vi "CopiaDeCopiaPAI.vi"() -> ()   [LabVIEW 2024]
uses:
  <vilib>/MakerHub/LINX/LMH-LINX.lvlib
  <vilib>/MakerHub/LINX/Public/Peripherals/Digital/Digital Read 1 Chan.vi
  <vilib>/MakerHub/LINX/Public/Peripherals/Digital/Digital Write 1 Chan.vi
  <vilib>/MakerHub/LINX/Public/Utilities/Open Serial.vi
panel:
  in  "Tab Control":enum32{"Inicio", "Sistema"}(tab)
  in  "Open Button 2":bool
  in  "Contraseña":string
  in  "Usuario":string
  out "Led 1":bool
  out "Led 2":bool
  out "Led 3":bool
  out "Led 4":bool
  out "Led 5":bool
  out "Pin2":dbl
  out "Pin3":dbl
  out "Pin4":dbl
  out "Pin5":dbl
  out "Pin6":dbl
  in  "Puerto Serial":refnum<visa-resource-name>="N/A"
  in  "Secuencia":dbl
  out "Contenido":dbl
  in  "Detener":bool
  in  "stop 4":bool
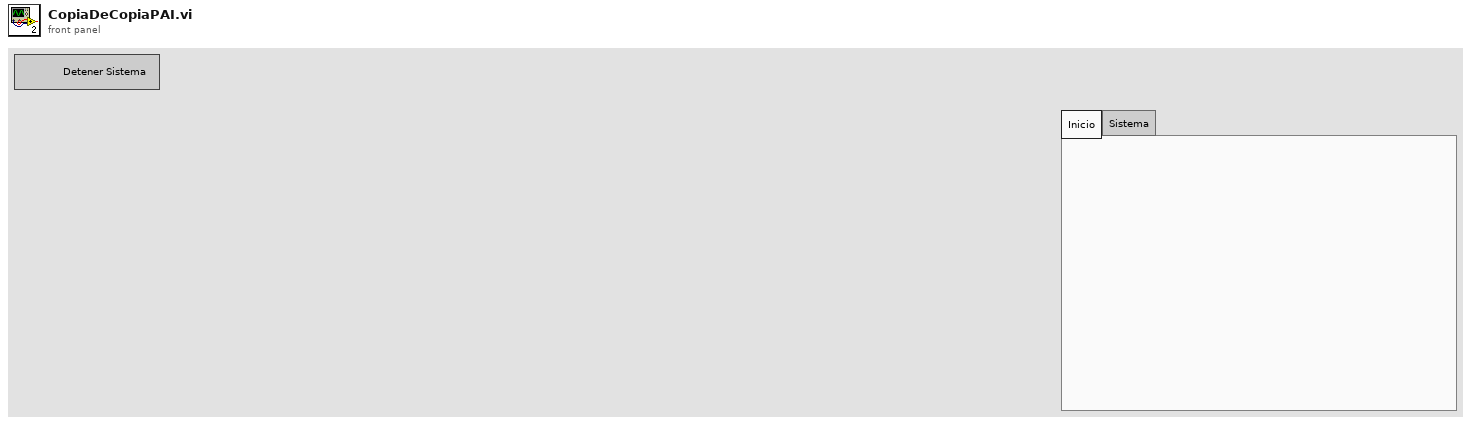
[diagram p1: front panel]
types:
  T1 = typedef "LMH-LINX.lvlib/LINX Ref.ctl" = cluster{"IO":T2, "Interface":T3, "LINX Device Config":T4}
  T2 = typedef "LMH-LINX.lvlib/Platform.ctl" = enum16{"Remote", "Local"}
  T3 = typedef "LMH-LINX.lvlib/Interface.ctl" = enum16{"Serial", "TCP"}
  T4 = typedef "LMH-LINX.lvlib/Device.lvlib/LINX Device Config.ctl" = cluster{"Interface":T3, "COM Port":refnum<visa-resource-name>, "TCP Configuration":T5, "Device Family":u8, "Device ID":u8, "Device Name":string, "TCP Ref":refnum<k5>, "Channels":T6}
  T5 = typedef "LMH-LINX.lvlib/Device.lvlib/TCP Config.ctl" = cluster{"IP Address":string, "Port":u16}
  T6 = typedef "LMH-LINX.lvlib/Channels.ctl" = cluster{"DI":u8[], "DO":u8[], "AI":u8[], "AO":u8[], "PWM":u8[], "QE":u8[], "UART":u8[], "I2C 2":u8[], "SPI":u8[], "CAN":u8[], "Servo":u8[], "AI Ref (V)":dbl, "AI Resolution (Bits)":u8, "AO Ref (V)":dbl, "AO Resolution (Bits)":u8}
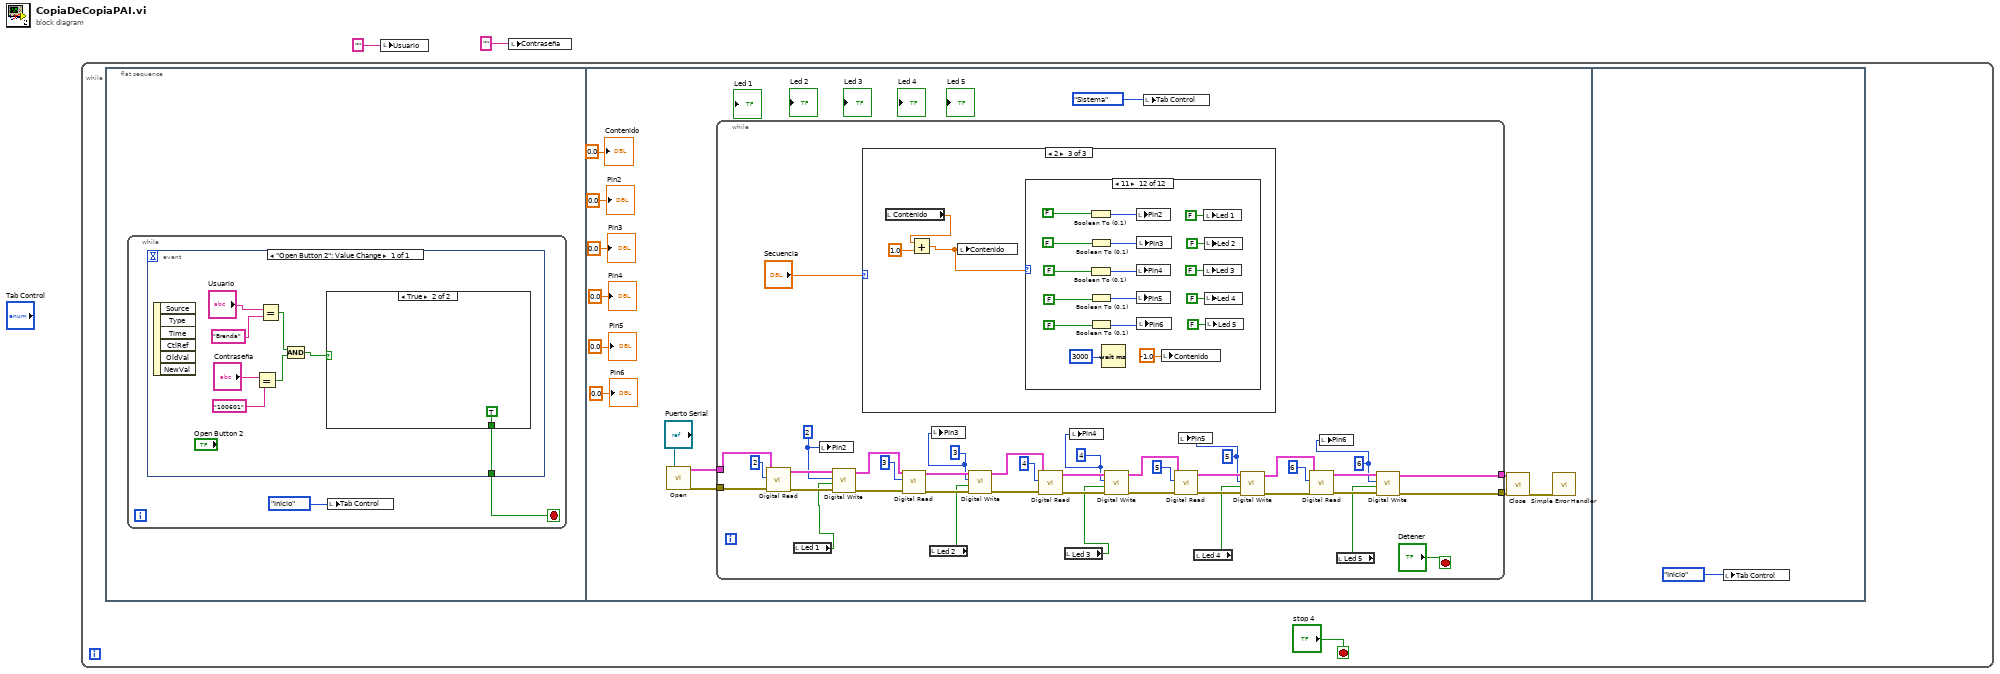
[diagram p0: block diagram]
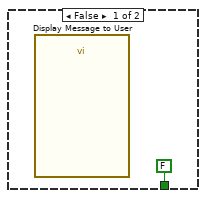
[diagram p2: hidden frame]
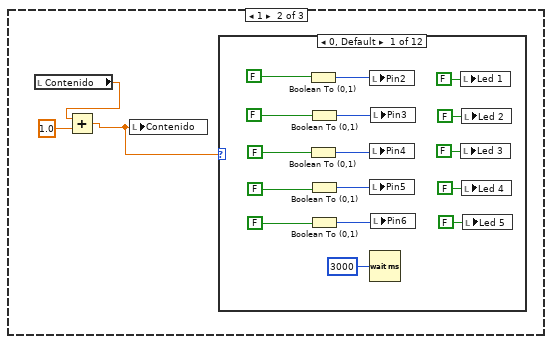
[diagram p4: hidden frame]
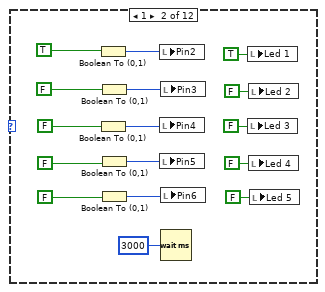
[diagram p5: hidden frame]
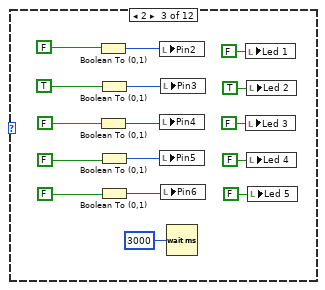
[diagram p6: hidden frame]
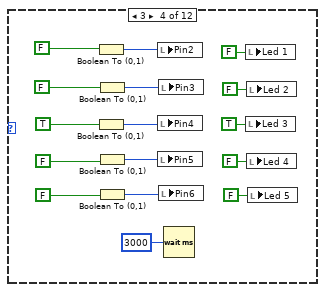
[diagram p7: hidden frame]
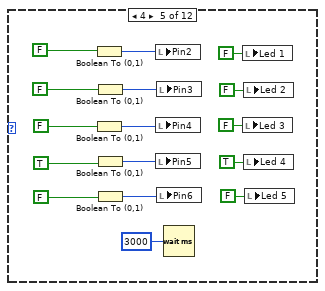
[diagram p8: hidden frame]
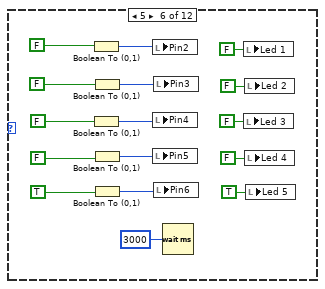
[diagram p9: hidden frame]
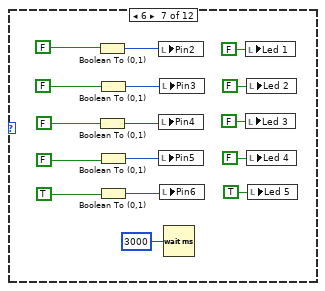
[diagram p10: hidden frame]
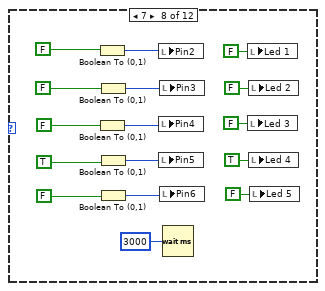
[diagram p11: hidden frame]
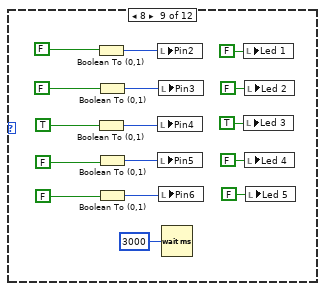
[diagram p12: hidden frame]
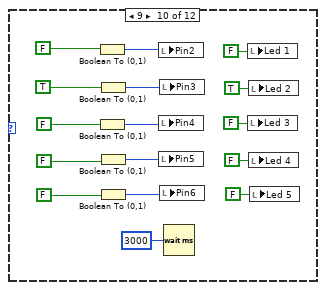
[diagram p13: hidden frame]
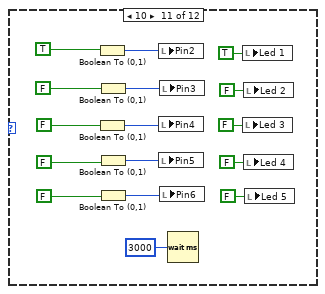
[diagram p14: hidden frame]
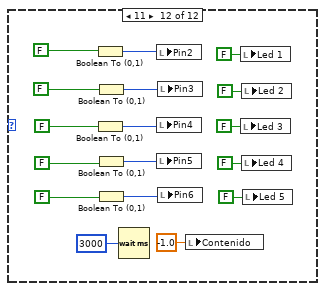
[diagram p15: hidden frame]
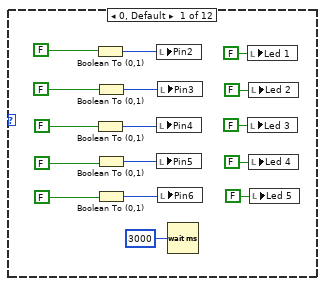
[diagram p16: hidden frame]
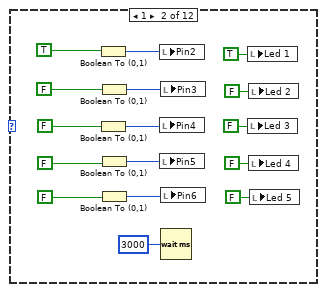
[diagram p17: hidden frame]
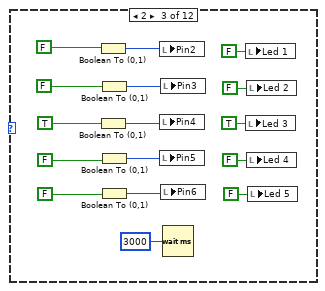
[diagram p18: hidden frame]
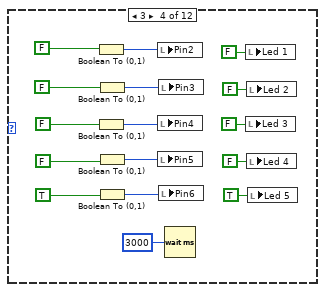
[diagram p19: hidden frame]
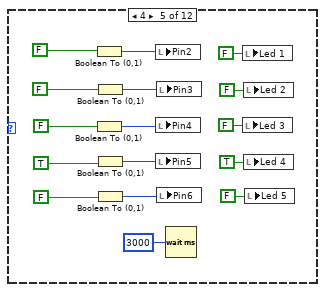
[diagram p20: hidden frame]
diagram:
  n1 = while {
    stop <- "stop 4" stop-if-true
    n2 = flat-sequence {
      frame #0 {
        n3 = while {
          stop <- w5 stop-if-true
          n4 = event shown="[0] \"Open Button 2\": Value Change" {
            selector: _ -> [_]
            dyn-events: _ -> [_]
            timeout: _ -> [_]
            tunnel: [w8] -> w5
            event "Open Button 2": Value Change {
              n5 = event-data() -> ()  [unwired: 1 in, 6 out]
              n6 = Equal?(x="Contraseña", y="100601") -> (x = y?=w10:bool)
              n7 = Equal?(x="Usuario", y="Brenda") -> (x = y?=w11:bool)
              n8 = And(x=w11, y=w10) -> (x .and. y?=w9:bool)
              n9 = case shown="True" w9 {
                tunnel: [FALSE TRUE] -> w8
                frame False {
                  n10 = call "Display Message to User"() -> ()  [unwired: 10 in, 2 out]
                }
                frame True {
                }
              }
            }
          }
          n11 = local write "Tab Control"(enum32{"Inicio", "Sistema"}."Inicio" ("Tab Control")) -> ()
        }
      }
      frame #1 {
        n12 = call-poly <vilib>:"Open.vi"("Serial Port"="Puerto Serial") -> ("Error Out"=w17:errorcluster, "LINX Resource"=w18:T1)  [unwired: 8 in, 1 out]
        n13 = while {
          tunnel: [w34] -> w20
          tunnel: [w33] -> w19
          tunnel: w18 -> [w32]
          tunnel: w17 -> [w31]
          stop <- "Detener" stop-if-true
          w35 = u8 6 ("DO Channel")
          w38 = u8 5 ("DO Channel")
          w39 = u8 4 ("DO Channel")
          w44 = u8 3 ("DO Channel")
          w42 = u8 2 ("DO Channel")
          n14 = call-poly <vilib>:"Digital Read.vi"("Error In"=w31, "DI Channel"=u8 2, "LINX Resource"=w32) -> ("Error Out"=w53:errorcluster, "LINX Resource"=w62:T1)  [unwired: 6 in, 1 out]
          n15 = local read "Led 1"() -> (w43:bool)
          n16 = local write "Pin2"(w42) -> ()
          n17 = call-poly <vilib>:"Digital Write.vi"("Error In"=w53, "Output Value"=w43, "DO Channel"=w42, "LINX Resource"=w62) -> ("Error Out"=w52:errorcluster, "LINX Resource"=w61:T1)  [unwired: 6 in]
          n18 = case shown="2" "Secuencia" {
            frame 0, Default {
            }
            frame 1 {
              n19 = local read "Contenido"() -> (w69:dbl)
              n20 = Add(x=w69, y=1.0) -> (x+y=w68:dbl)
              n21 = local write "Contenido"(w68) -> ()
              n22 = case shown="0, Default" w68 {
                frame 0, Default {
                  n23 = Boolean To (0,1)(Boolean=FALSE) -> (0, 1=w86:i16)
                  n24 = Boolean To (0,1)(Boolean=FALSE) -> (0, 1=w84:i16)
                  n25 = Boolean To (0,1)(Boolean=FALSE) -> (0, 1=w85:i16)
                  n26 = Boolean To (0,1)(Boolean=FALSE) -> (0, 1=w83:i16)
                  n27 = Boolean To (0,1)(Boolean=FALSE) -> (0, 1=w82:i16)
                  n28 = local write "Pin2"(w86) -> ()
                  n29 = local write "Pin4"(w84) -> ()
                  n30 = local write "Pin5"(w83) -> ()
                  n31 = Wait (ms)(milliseconds to wait=u32 3000 ("millisecond timer value")) -> ()  [unwired: 1 out]
                  n32 = local write "Pin3"(w85) -> ()
                  n33 = local write "Pin6"(w82) -> ()
                  n34 = local write "Led 1"(FALSE ("Led 1")) -> ()
                  n35 = local write "Led 3"(FALSE ("Led 3")) -> ()
                  n36 = local write "Led 2"(FALSE ("Led 2")) -> ()
                  n37 = local write "Led 4"(FALSE ("Led 4")) -> ()
                  n38 = local write "Led 5"(FALSE ("Led 5")) -> ()
                }
                frame 1 {
                  n39 = Boolean To (0,1)(Boolean=TRUE) -> (0, 1=w101:i16)
                  n40 = Boolean To (0,1)(Boolean=FALSE) -> (0, 1=w97:i16)
                  n41 = Boolean To (0,1)(Boolean=FALSE) -> (0, 1=w99:i16)
                  n42 = Boolean To (0,1)(Boolean=FALSE) -> (0, 1=w95:i16)
                  n43 = Boolean To (0,1)(Boolean=FALSE) -> (0, 1=w93:i16)
                  n44 = local write "Pin2"(w101) -> ()
                  n45 = local write "Pin4"(w97) -> ()
                  n46 = local write "Pin5"(w95) -> ()
                  n47 = local write "Pin3"(w99) -> ()
                  n48 = local write "Pin6"(w93) -> ()
                  n49 = Wait (ms)(milliseconds to wait=u32 3000 ("millisecond timer value")) -> ()  [unwired: 1 out]
                  n50 = local write "Led 1"(TRUE ("Led 1")) -> ()
                  n51 = local write "Led 3"(FALSE ("Led 3")) -> ()
                  n52 = local write "Led 2"(FALSE ("Led 2")) -> ()
                  n53 = local write "Led 4"(FALSE ("Led 4")) -> ()
                  n54 = local write "Led 5"(FALSE ("Led 5")) -> ()
                }
                frame 2 {
                  n55 = Boolean To (0,1)(Boolean=FALSE) -> (0, 1=w118:i16)
                  n56 = Boolean To (0,1)(Boolean=FALSE) -> (0, 1=w116:i16)
                  n57 = Boolean To (0,1)(Boolean=TRUE) -> (0, 1=w117:i16)
                  n58 = Boolean To (0,1)(Boolean=FALSE) -> (0, 1=w115:i16)
                  n59 = Boolean To (0,1)(Boolean=FALSE) -> (0, 1=w114:i16)
                  n60 = local write "Pin2"(w118) -> ()
                  n61 = local write "Pin4"(w116) -> ()
                  n62 = local write "Pin5"(w115) -> ()
                  n63 = local write "Pin3"(w117) -> ()
                  n64 = local write "Pin6"(w114) -> ()
                  n65 = Wait (ms)(milliseconds to wait=u32 3000 ("millisecond timer value")) -> ()  [unwired: 1 out]
                  n66 = local write "Led 1"(FALSE ("Led 1")) -> ()
                  n67 = local write "Led 3"(FALSE ("Led 3")) -> ()
                  n68 = local write "Led 2"(TRUE ("Led 2")) -> ()
                  n69 = local write "Led 4"(FALSE ("Led 4")) -> ()
                  n70 = local write "Led 5"(FALSE ("Led 5")) -> ()
                }
                frame 3 {
                  n71 = Boolean To (0,1)(Boolean=FALSE) -> (0, 1=w134:i16)
                  n72 = Boolean To (0,1)(Boolean=TRUE) -> (0, 1=w132:i16)
                  n73 = Boolean To (0,1)(Boolean=FALSE) -> (0, 1=w133:i16)
                  n74 = Boolean To (0,1)(Boolean=FALSE) -> (0, 1=w131:i16)
                  n75 = Boolean To (0,1)(Boolean=FALSE) -> (0, 1=w130:i16)
                  n76 = local write "Pin2"(w134) -> ()
                  n77 = local write "Pin4"(w132) -> ()
                  n78 = local write "Pin5"(w131) -> ()
                  n79 = local write "Pin3"(w133) -> ()
                  n80 = local write "Pin6"(w130) -> ()
                  n81 = Wait (ms)(milliseconds to wait=u32 3000 ("millisecond timer value")) -> ()  [unwired: 1 out]
                  n82 = local write "Led 1"(FALSE ("Led 1")) -> ()
                  n83 = local write "Led 3"(TRUE ("Led 3")) -> ()
                  n84 = local write "Led 2"(FALSE ("Led 2")) -> ()
                  n85 = local write "Led 4"(FALSE ("Led 4")) -> ()
                  n86 = local write "Led 5"(FALSE ("Led 5")) -> ()
                }
                frame 4 {
                  n87 = Boolean To (0,1)(Boolean=FALSE) -> (0, 1=w150:i16)
                  n88 = Boolean To (0,1)(Boolean=FALSE) -> (0, 1=w148:i16)
                  n89 = Boolean To (0,1)(Boolean=FALSE) -> (0, 1=w149:i16)
                  n90 = Boolean To (0,1)(Boolean=TRUE) -> (0, 1=w147:i16)
                  n91 = Boolean To (0,1)(Boolean=FALSE) -> (0, 1=w146:i16)
                  n92 = local write "Pin2"(w150) -> ()
                  n93 = local write "Pin4"(w148) -> ()
                  n94 = local write "Pin5"(w147) -> ()
                  n95 = local write "Pin3"(w149) -> ()
                  n96 = local write "Pin6"(w146) -> ()
                  n97 = Wait (ms)(milliseconds to wait=u32 3000 ("millisecond timer value")) -> ()  [unwired: 1 out]
                  n98 = local write "Led 1"(FALSE ("Led 1")) -> ()
                  n99 = local write "Led 3"(FALSE ("Led 3")) -> ()
                  n100 = local write "Led 2"(FALSE ("Led 2")) -> ()
                  n101 = local write "Led 4"(TRUE ("Led 4")) -> ()
                  n102 = local write "Led 5"(FALSE ("Led 5")) -> ()
                }
                frame 5 {
                  n103 = Boolean To (0,1)(Boolean=FALSE) -> (0, 1=w166:i16)
                  n104 = Boolean To (0,1)(Boolean=FALSE) -> (0, 1=w164:i16)
                  n105 = Boolean To (0,1)(Boolean=FALSE) -> (0, 1=w165:i16)
                  n106 = Boolean To (0,1)(Boolean=FALSE) -> (0, 1=w163:i16)
                  n107 = Boolean To (0,1)(Boolean=TRUE) -> (0, 1=w162:i16)
                  n108 = local write "Pin2"(w166) -> ()
                  n109 = local write "Pin4"(w164) -> ()
                  n110 = local write "Pin5"(w163) -> ()
                  n111 = local write "Pin3"(w165) -> ()
                  n112 = local write "Pin6"(w162) -> ()
                  n113 = Wait (ms)(milliseconds to wait=u32 3000 ("millisecond timer value")) -> ()  [unwired: 1 out]
                  n114 = local write "Led 1"(FALSE ("Led 1")) -> ()
                  n115 = local write "Led 3"(FALSE ("Led 3")) -> ()
                  n116 = local write "Led 2"(FALSE ("Led 2")) -> ()
                  n117 = local write "Led 4"(FALSE ("Led 4")) -> ()
                  n118 = local write "Led 5"(TRUE ("Led 5")) -> ()
                }
                frame 6 {
                  n119 = Boolean To (0,1)(Boolean=FALSE) -> (0, 1=w182:i16)
                  n120 = Boolean To (0,1)(Boolean=FALSE) -> (0, 1=w180:i16)
                  n121 = Boolean To (0,1)(Boolean=FALSE) -> (0, 1=w181:i16)
                  n122 = Boolean To (0,1)(Boolean=FALSE) -> (0, 1=w179:i16)
                  n123 = Boolean To (0,1)(Boolean=TRUE) -> (0, 1=w178:i16)
                  n124 = local write "Pin2"(w182) -> ()
                  n125 = local write "Pin4"(w180) -> ()
                  n126 = local write "Pin5"(w179) -> ()
                  n127 = local write "Pin3"(w181) -> ()
                  n128 = local write "Pin6"(w178) -> ()
                  n129 = Wait (ms)(milliseconds to wait=u32 3000 ("millisecond timer value")) -> ()  [unwired: 1 out]
                  n130 = local write "Led 1"(FALSE ("Led 1")) -> ()
                  n131 = local write "Led 3"(FALSE ("Led 3")) -> ()
                  n132 = local write "Led 2"(FALSE ("Led 2")) -> ()
                  n133 = local write "Led 4"(FALSE ("Led 4")) -> ()
                  n134 = local write "Led 5"(TRUE ("Led 5")) -> ()
                }
                frame 7 {
                  n135 = Boolean To (0,1)(Boolean=FALSE) -> (0, 1=w198:i16)
                  n136 = Boolean To (0,1)(Boolean=FALSE) -> (0, 1=w196:i16)
                  n137 = Boolean To (0,1)(Boolean=FALSE) -> (0, 1=w197:i16)
                  n138 = Boolean To (0,1)(Boolean=TRUE) -> (0, 1=w195:i16)
                  n139 = Boolean To (0,1)(Boolean=FALSE) -> (0, 1=w194:i16)
                  n140 = local write "Pin2"(w198) -> ()
                  n141 = local write "Pin4"(w196) -> ()
                  n142 = local write "Pin5"(w195) -> ()
                  n143 = local write "Pin3"(w197) -> ()
                  n144 = local write "Pin6"(w194) -> ()
                  n145 = Wait (ms)(milliseconds to wait=u32 3000 ("millisecond timer value")) -> ()  [unwired: 1 out]
                  n146 = local write "Led 1"(FALSE ("Led 1")) -> ()
                  n147 = local write "Led 3"(FALSE ("Led 3")) -> ()
                  n148 = local write "Led 2"(FALSE ("Led 2")) -> ()
                  n149 = local write "Led 4"(TRUE ("Led 4")) -> ()
                  n150 = local write "Led 5"(FALSE ("Led 5")) -> ()
                }
                frame 8 {
                  n151 = Boolean To (0,1)(Boolean=FALSE) -> (0, 1=w214:i16)
                  n152 = Boolean To (0,1)(Boolean=TRUE) -> (0, 1=w212:i16)
                  n153 = Boolean To (0,1)(Boolean=FALSE) -> (0, 1=w213:i16)
                  n154 = Boolean To (0,1)(Boolean=FALSE) -> (0, 1=w211:i16)
                  n155 = Boolean To (0,1)(Boolean=FALSE) -> (0, 1=w210:i16)
                  n156 = local write "Pin2"(w214) -> ()
                  n157 = local write "Pin4"(w212) -> ()
                  n158 = local write "Pin5"(w211) -> ()
                  n159 = local write "Pin3"(w213) -> ()
                  n160 = local write "Pin6"(w210) -> ()
                  n161 = Wait (ms)(milliseconds to wait=u32 3000 ("millisecond timer value")) -> ()  [unwired: 1 out]
                  n162 = local write "Led 1"(FALSE ("Led 1")) -> ()
                  n163 = local write "Led 3"(TRUE ("Led 3")) -> ()
                  n164 = local write "Led 2"(FALSE ("Led 2")) -> ()
                  n165 = local write "Led 4"(FALSE ("Led 4")) -> ()
                  n166 = local write "Led 5"(FALSE ("Led 5")) -> ()
                }
                frame 9 {
                  n167 = Boolean To (0,1)(Boolean=FALSE) -> (0, 1=w230:i16)
                  n168 = Boolean To (0,1)(Boolean=FALSE) -> (0, 1=w228:i16)
                  n169 = Boolean To (0,1)(Boolean=TRUE) -> (0, 1=w229:i16)
                  n170 = Boolean To (0,1)(Boolean=FALSE) -> (0, 1=w227:i16)
                  n171 = Boolean To (0,1)(Boolean=FALSE) -> (0, 1=w226:i16)
                  n172 = local write "Pin2"(w230) -> ()
                  n173 = local write "Pin4"(w228) -> ()
                  n174 = local write "Pin5"(w227) -> ()
                  n175 = local write "Pin3"(w229) -> ()
                  n176 = local write "Pin6"(w226) -> ()
                  n177 = Wait (ms)(milliseconds to wait=u32 3000 ("millisecond timer value")) -> ()  [unwired: 1 out]
                  n178 = local write "Led 1"(FALSE ("Led 1")) -> ()
                  n179 = local write "Led 3"(FALSE ("Led 3")) -> ()
                  n180 = local write "Led 2"(TRUE ("Led 2")) -> ()
                  n181 = local write "Led 4"(FALSE ("Led 4")) -> ()
                  n182 = local write "Led 5"(FALSE ("Led 5")) -> ()
                }
                frame 10 {
                  n183 = Boolean To (0,1)(Boolean=TRUE) -> (0, 1=w246:i16)
                  n184 = Boolean To (0,1)(Boolean=FALSE) -> (0, 1=w244:i16)
                  n185 = Boolean To (0,1)(Boolean=FALSE) -> (0, 1=w245:i16)
                  n186 = Boolean To (0,1)(Boolean=FALSE) -> (0, 1=w243:i16)
                  n187 = Boolean To (0,1)(Boolean=FALSE) -> (0, 1=w242:i16)
                  n188 = local write "Pin2"(w246) -> ()
                  n189 = local write "Pin4"(w244) -> ()
                  n190 = local write "Pin5"(w243) -> ()
                  n191 = local write "Pin3"(w245) -> ()
                  n192 = local write "Pin6"(w242) -> ()
                  n193 = Wait (ms)(milliseconds to wait=u32 3000 ("millisecond timer value")) -> ()  [unwired: 1 out]
                  n194 = local write "Led 1"(TRUE ("Led 1")) -> ()
                  n195 = local write "Led 3"(FALSE ("Led 3")) -> ()
                  n196 = local write "Led 2"(FALSE ("Led 2")) -> ()
                  n197 = local write "Led 4"(FALSE ("Led 4")) -> ()
                  n198 = local write "Led 5"(FALSE ("Led 5")) -> ()
                }
                frame 11 {
                  n199 = Boolean To (0,1)(Boolean=FALSE) -> (0, 1=w263:i16)
                  n200 = Boolean To (0,1)(Boolean=FALSE) -> (0, 1=w261:i16)
                  n201 = Boolean To (0,1)(Boolean=FALSE) -> (0, 1=w262:i16)
                  n202 = Boolean To (0,1)(Boolean=FALSE) -> (0, 1=w260:i16)
                  n203 = Boolean To (0,1)(Boolean=FALSE) -> (0, 1=w259:i16)
                  n204 = Wait (ms)(milliseconds to wait=u32 3000 ("millisecond timer value")) -> ()  [unwired: 1 out]
                  n205 = local write "Pin2"(w263) -> ()
                  n206 = local write "Pin4"(w261) -> ()
                  n207 = local write "Pin5"(w260) -> ()
                  n208 = local write "Pin3"(w262) -> ()
                  n209 = local write "Pin6"(w259) -> ()
                  n210 = local write "Contenido"(-1.0 ("Contenido")) -> ()
                  n211 = local write "Led 1"(FALSE ("Led 1")) -> ()
                  n212 = local write "Led 3"(FALSE ("Led 3")) -> ()
                  n213 = local write "Led 2"(FALSE ("Led 2")) -> ()
                  n214 = local write "Led 4"(FALSE ("Led 4")) -> ()
                  n215 = local write "Led 5"(FALSE ("Led 5")) -> ()
                }
              }
            }
            frame 2 {
              n216 = local read "Contenido"() -> (w266:dbl)
              n217 = Add(x=w266, y=1.0) -> (x+y=w265:dbl)
              n218 = local write "Contenido"(w265) -> ()
              n219 = case shown="11" w265 {
                frame 0, Default {
                  n220 = Boolean To (0,1)(Boolean=FALSE) -> (0, 1=w282:i16)
                  n221 = Boolean To (0,1)(Boolean=FALSE) -> (0, 1=w280:i16)
                  n222 = Boolean To (0,1)(Boolean=FALSE) -> (0, 1=w281:i16)
                  n223 = Boolean To (0,1)(Boolean=FALSE) -> (0, 1=w279:i16)
                  n224 = Boolean To (0,1)(Boolean=FALSE) -> (0, 1=w278:i16)
                  n225 = local write "Pin2"(w282) -> ()
                  n226 = local write "Pin4"(w280) -> ()
                  n227 = local write "Pin5"(w279) -> ()
                  n228 = local write "Pin3"(w281) -> ()
                  n229 = local write "Pin6"(w278) -> ()
                  n230 = Wait (ms)(milliseconds to wait=u32 3000 ("millisecond timer value")) -> ()  [unwired: 1 out]
                  n231 = local write "Led 1"(FALSE ("Led 1")) -> ()
                  n232 = local write "Led 3"(FALSE ("Led 3")) -> ()
                  n233 = local write "Led 2"(FALSE ("Led 2")) -> ()
                  n234 = local write "Led 4"(FALSE ("Led 4")) -> ()
                  n235 = local write "Led 5"(FALSE ("Led 5")) -> ()
                }
                frame 1 {
                  n236 = Boolean To (0,1)(Boolean=TRUE) -> (0, 1=w297:i16)
                  n237 = Boolean To (0,1)(Boolean=FALSE) -> (0, 1=w293:i16)
                  n238 = Boolean To (0,1)(Boolean=FALSE) -> (0, 1=w295:i16)
                  n239 = Boolean To (0,1)(Boolean=FALSE) -> (0, 1=w291:i16)
                  n240 = Boolean To (0,1)(Boolean=FALSE) -> (0, 1=w289:i16)
                  n241 = local write "Pin2"(w297) -> ()
                  n242 = local write "Pin4"(w293) -> ()
                  n243 = local write "Pin5"(w291) -> ()
                  n244 = local write "Pin3"(w295) -> ()
                  n245 = local write "Pin6"(w289) -> ()
                  n246 = Wait (ms)(milliseconds to wait=u32 3000 ("millisecond timer value")) -> ()  [unwired: 1 out]
                  n247 = local write "Led 1"(TRUE ("Led 1")) -> ()
                  n248 = local write "Led 3"(FALSE ("Led 3")) -> ()
                  n249 = local write "Led 2"(FALSE ("Led 2")) -> ()
                  n250 = local write "Led 4"(FALSE ("Led 4")) -> ()
                  n251 = local write "Led 5"(FALSE ("Led 5")) -> ()
                }
                frame 2 {
                  n252 = Boolean To (0,1)(Boolean=FALSE) -> (0, 1=w314:i16)
                  n253 = Boolean To (0,1)(Boolean=TRUE) -> (0, 1=w312:i16)
                  n254 = Boolean To (0,1)(Boolean=FALSE) -> (0, 1=w313:i16)
                  n255 = Boolean To (0,1)(Boolean=FALSE) -> (0, 1=w311:i16)
                  n256 = Boolean To (0,1)(Boolean=FALSE) -> (0, 1=w310:i16)
                  n257 = local write "Pin2"(w314) -> ()
                  n258 = local write "Pin4"(w312) -> ()
                  n259 = local write "Pin5"(w311) -> ()
                  n260 = local write "Pin3"(w313) -> ()
                  n261 = local write "Pin6"(w310) -> ()
                  n262 = Wait (ms)(milliseconds to wait=u32 3000 ("millisecond timer value")) -> ()  [unwired: 1 out]
                  n263 = local write "Led 1"(FALSE ("Led 1")) -> ()
                  n264 = local write "Led 3"(TRUE ("Led 3")) -> ()
                  n265 = local write "Led 2"(FALSE ("Led 2")) -> ()
                  n266 = local write "Led 4"(FALSE ("Led 4")) -> ()
                  n267 = local write "Led 5"(FALSE ("Led 5")) -> ()
                }
                frame 3 {
                  n268 = Boolean To (0,1)(Boolean=FALSE) -> (0, 1=w330:i16)
                  n269 = Boolean To (0,1)(Boolean=FALSE) -> (0, 1=w328:i16)
                  n270 = Boolean To (0,1)(Boolean=FALSE) -> (0, 1=w329:i16)
                  n271 = Boolean To (0,1)(Boolean=FALSE) -> (0, 1=w327:i16)
                  n272 = Boolean To (0,1)(Boolean=TRUE) -> (0, 1=w326:i16)
                  n273 = local write "Pin2"(w330) -> ()
                  n274 = local write "Pin4"(w328) -> ()
                  n275 = local write "Pin5"(w327) -> ()
                  n276 = local write "Pin3"(w329) -> ()
                  n277 = local write "Pin6"(w326) -> ()
                  n278 = Wait (ms)(milliseconds to wait=u32 3000 ("millisecond timer value")) -> ()  [unwired: 1 out]
                  n279 = local write "Led 1"(FALSE ("Led 1")) -> ()
                  n280 = local write "Led 3"(FALSE ("Led 3")) -> ()
                  n281 = local write "Led 2"(FALSE ("Led 2")) -> ()
                  n282 = local write "Led 4"(FALSE ("Led 4")) -> ()
                  n283 = local write "Led 5"(TRUE ("Led 5")) -> ()
                }
                frame 4 {
                  n284 = Boolean To (0,1)(Boolean=FALSE) -> (0, 1=w346:i16)
                  n285 = Boolean To (0,1)(Boolean=FALSE) -> (0, 1=w344:i16)
                  n286 = Boolean To (0,1)(Boolean=FALSE) -> (0, 1=w345:i16)
                  n287 = Boolean To (0,1)(Boolean=TRUE) -> (0, 1=w343:i16)
                  n288 = Boolean To (0,1)(Boolean=FALSE) -> (0, 1=w342:i16)
                  n289 = local write "Pin2"(w346) -> ()
                  n290 = local write "Pin4"(w344) -> ()
                  n291 = local write "Pin5"(w343) -> ()
                  n292 = local write "Pin3"(w345) -> ()
                  n293 = local write "Pin6"(w342) -> ()
                  n294 = Wait (ms)(milliseconds to wait=u32 3000 ("millisecond timer value")) -> ()  [unwired: 1 out]
                  n295 = local write "Led 1"(FALSE ("Led 1")) -> ()
                  n296 = local write "Led 3"(FALSE ("Led 3")) -> ()
                  n297 = local write "Led 2"(FALSE ("Led 2")) -> ()
                  n298 = local write "Led 4"(TRUE ("Led 4")) -> ()
                  n299 = local write "Led 5"(FALSE ("Led 5")) -> ()
                }
                frame 5 {
                  n300 = Boolean To (0,1)(Boolean=FALSE) -> (0, 1=w362:i16)
                  n301 = Boolean To (0,1)(Boolean=FALSE) -> (0, 1=w360:i16)
                  n302 = Boolean To (0,1)(Boolean=TRUE) -> (0, 1=w361:i16)
                  n303 = Boolean To (0,1)(Boolean=FALSE) -> (0, 1=w359:i16)
                  n304 = Boolean To (0,1)(Boolean=FALSE) -> (0, 1=w358:i16)
                  n305 = local write "Pin2"(w362) -> ()
                  n306 = local write "Pin4"(w360) -> ()
                  n307 = local write "Pin5"(w359) -> ()
                  n308 = local write "Pin3"(w361) -> ()
                  n309 = local write "Pin6"(w358) -> ()
                  n310 = Wait (ms)(milliseconds to wait=u32 3000 ("millisecond timer value")) -> ()  [unwired: 1 out]
                  n311 = local write "Led 1"(FALSE ("Led 1")) -> ()
                  n312 = local write "Led 3"(FALSE ("Led 3")) -> ()
                  n313 = local write "Led 2"(TRUE ("Led 2")) -> ()
                  n314 = local write "Led 4"(FALSE ("Led 4")) -> ()
                  n315 = local write "Led 5"(FALSE ("Led 5")) -> ()
                }
                frame 6 {
                  n316 = Boolean To (0,1)(Boolean=FALSE) -> (0, 1=w378:i16)
                  n317 = Boolean To (0,1)(Boolean=FALSE) -> (0, 1=w376:i16)
                  n318 = Boolean To (0,1)(Boolean=TRUE) -> (0, 1=w377:i16)
                  n319 = Boolean To (0,1)(Boolean=FALSE) -> (0, 1=w375:i16)
                  n320 = Boolean To (0,1)(Boolean=FALSE) -> (0, 1=w374:i16)
                  n321 = local write "Pin2"(w378) -> ()
                  n322 = local write "Pin4"(w376) -> ()
                  n323 = local write "Pin5"(w375) -> ()
                  n324 = local write "Pin3"(w377) -> ()
                  n325 = local write "Pin6"(w374) -> ()
                  n326 = Wait (ms)(milliseconds to wait=u32 3000 ("millisecond timer value")) -> ()  [unwired: 1 out]
                  n327 = local write "Led 1"(FALSE ("Led 1")) -> ()
                  n328 = local write "Led 3"(FALSE ("Led 3")) -> ()
                  n329 = local write "Led 2"(TRUE ("Led 2")) -> ()
                  n330 = local write "Led 4"(FALSE ("Led 4")) -> ()
                  n331 = local write "Led 5"(FALSE ("Led 5")) -> ()
                }
                frame 7 {
                  n332 = Boolean To (0,1)(Boolean=FALSE) -> (0, 1=w394:i16)
                  n333 = Boolean To (0,1)(Boolean=FALSE) -> (0, 1=w392:i16)
                  n334 = Boolean To (0,1)(Boolean=FALSE) -> (0, 1=w393:i16)
                  n335 = Boolean To (0,1)(Boolean=TRUE) -> (0, 1=w391:i16)
                  n336 = Boolean To (0,1)(Boolean=FALSE) -> (0, 1=w390:i16)
                  n337 = local write "Pin2"(w394) -> ()
                  n338 = local write "Pin4"(w392) -> ()
                  n339 = local write "Pin5"(w391) -> ()
                  n340 = local write "Pin3"(w393) -> ()
                  n341 = local write "Pin6"(w390) -> ()
                  n342 = Wait (ms)(milliseconds to wait=u32 3000 ("millisecond timer value")) -> ()  [unwired: 1 out]
                  n343 = local write "Led 1"(FALSE ("Led 1")) -> ()
                  n344 = local write "Led 3"(FALSE ("Led 3")) -> ()
                  n345 = local write "Led 2"(FALSE ("Led 2")) -> ()
                  n346 = local write "Led 4"(TRUE ("Led 4")) -> ()
                  n347 = local write "Led 5"(FALSE ("Led 5")) -> ()
                }
                frame 8 {
                  n348 = Boolean To (0,1)(Boolean=FALSE) -> (0, 1=w410:i16)
                  n349 = Boolean To (0,1)(Boolean=TRUE) -> (0, 1=w408:i16)
                  n350 = Boolean To (0,1)(Boolean=FALSE) -> (0, 1=w409:i16)
                  n351 = Boolean To (0,1)(Boolean=FALSE) -> (0, 1=w407:i16)
                  n352 = Boolean To (0,1)(Boolean=FALSE) -> (0, 1=w406:i16)
                  n353 = local write "Pin2"(w410) -> ()
                  n354 = local write "Pin4"(w408) -> ()
                  n355 = local write "Pin5"(w407) -> ()
                  n356 = local write "Pin3"(w409) -> ()
                  n357 = local write "Pin6"(w406) -> ()
                  n358 = Wait (ms)(milliseconds to wait=u32 3000 ("millisecond timer value")) -> ()  [unwired: 1 out]
                  n359 = local write "Led 1"(FALSE ("Led 1")) -> ()
                  n360 = local write "Led 3"(TRUE ("Led 3")) -> ()
                  n361 = local write "Led 2"(FALSE ("Led 2")) -> ()
                  n362 = local write "Led 4"(FALSE ("Led 4")) -> ()
                  n363 = local write "Led 5"(FALSE ("Led 5")) -> ()
                }
                frame 9 {
                  n364 = Boolean To (0,1)(Boolean=FALSE) -> (0, 1=w426:i16)
                  n365 = Boolean To (0,1)(Boolean=FALSE) -> (0, 1=w424:i16)
                  n366 = Boolean To (0,1)(Boolean=FALSE) -> (0, 1=w425:i16)
                  n367 = Boolean To (0,1)(Boolean=FALSE) -> (0, 1=w423:i16)
                  n368 = Boolean To (0,1)(Boolean=TRUE) -> (0, 1=w422:i16)
                  n369 = local write "Pin2"(w426) -> ()
                  n370 = local write "Pin4"(w424) -> ()
                  n371 = local write "Pin5"(w423) -> ()
                  n372 = local write "Pin3"(w425) -> ()
                  n373 = local write "Pin6"(w422) -> ()
                  n374 = Wait (ms)(milliseconds to wait=u32 3000 ("millisecond timer value")) -> ()  [unwired: 1 out]
                  n375 = local write "Led 1"(FALSE ("Led 1")) -> ()
                  n376 = local write "Led 3"(FALSE ("Led 3")) -> ()
                  n377 = local write "Led 2"(FALSE ("Led 2")) -> ()
                  n378 = local write "Led 4"(FALSE ("Led 4")) -> ()
                  n379 = local write "Led 5"(TRUE ("Led 5")) -> ()
                }
                frame 10 {
                  n380 = Boolean To (0,1)(Boolean=TRUE) -> (0, 1=w442:i16)
                  n381 = Boolean To (0,1)(Boolean=FALSE) -> (0, 1=w440:i16)
                  n382 = Boolean To (0,1)(Boolean=FALSE) -> (0, 1=w441:i16)
                  n383 = Boolean To (0,1)(Boolean=FALSE) -> (0, 1=w439:i16)
                  n384 = Boolean To (0,1)(Boolean=FALSE) -> (0, 1=w438:i16)
                  n385 = local write "Pin2"(w442) -> ()
                  n386 = local write "Pin4"(w440) -> ()
                  n387 = local write "Pin5"(w439) -> ()
                  n388 = local write "Pin3"(w441) -> ()
                  n389 = local write "Pin6"(w438) -> ()
                  n390 = Wait (ms)(milliseconds to wait=u32 3000 ("millisecond timer value")) -> ()  [unwired: 1 out]
                  n391 = local write "Led 1"(TRUE ("Led 1")) -> ()
                  n392 = local write "Led 3"(FALSE ("Led 3")) -> ()
                  n393 = local write "Led 2"(FALSE ("Led 2")) -> ()
                  n394 = local write "Led 4"(FALSE ("Led 4")) -> ()
                  n395 = local write "Led 5"(FALSE ("Led 5")) -> ()
                }
                frame 11 {
                  n396 = Boolean To (0,1)(Boolean=FALSE) -> (0, 1=w459:i16)
                  n397 = Boolean To (0,1)(Boolean=FALSE) -> (0, 1=w457:i16)
                  n398 = Boolean To (0,1)(Boolean=FALSE) -> (0, 1=w458:i16)
                  n399 = Boolean To (0,1)(Boolean=FALSE) -> (0, 1=w456:i16)
                  n400 = Boolean To (0,1)(Boolean=FALSE) -> (0, 1=w455:i16)
                  n401 = Wait (ms)(milliseconds to wait=u32 3000 ("millisecond timer value")) -> ()  [unwired: 1 out]
                  n402 = local write "Pin2"(w459) -> ()
                  n403 = local write "Pin4"(w457) -> ()
                  n404 = local write "Pin5"(w456) -> ()
                  n405 = local write "Pin3"(w458) -> ()
                  n406 = local write "Pin6"(w455) -> ()
                  n407 = local write "Contenido"(-1.0 ("Contenido")) -> ()
                  n408 = local write "Led 1"(FALSE ("Led 1")) -> ()
                  n409 = local write "Led 3"(FALSE ("Led 3")) -> ()
                  n410 = local write "Led 2"(FALSE ("Led 2")) -> ()
                  n411 = local write "Led 4"(FALSE ("Led 4")) -> ()
                  n412 = local write "Led 5"(FALSE ("Led 5")) -> ()
                }
              }
            }
          }
          n413 = call-poly <vilib>:"Digital Read.vi"("Error In"=w52, "DI Channel"=u8 3, "LINX Resource"=w61) -> ("Error Out"=w51:errorcluster, "LINX Resource"=w60:T1)  [unwired: 6 in, 1 out]
          n414 = local read "Led 2"() -> (w41:bool)
          n415 = local write "Pin3"(w44) -> ()
          n416 = call-poly <vilib>:"Digital Write.vi"("Error In"=w51, "Output Value"=w41, "DO Channel"=w44, "LINX Resource"=w60) -> ("Error Out"=w50:errorcluster, "LINX Resource"=w59:T1)  [unwired: 6 in]
          n417 = call-poly <vilib>:"Digital Read.vi"("Error In"=w50, "DI Channel"=u8 4, "LINX Resource"=w59) -> ("Error Out"=w49:errorcluster, "LINX Resource"=w58:T1)  [unwired: 6 in, 1 out]
          n418 = local read "Led 3"() -> (w40:bool)
          n419 = local write "Pin4"(w39) -> ()
          n420 = call-poly <vilib>:"Digital Write.vi"("Error In"=w49, "Output Value"=w40, "DO Channel"=w39, "LINX Resource"=w58) -> ("Error Out"=w48:errorcluster, "LINX Resource"=w57:T1)  [unwired: 6 in]
          n421 = call-poly <vilib>:"Digital Read.vi"("Error In"=w48, "DI Channel"=u8 5, "LINX Resource"=w57) -> ("Error Out"=w47:errorcluster, "LINX Resource"=w56:T1)  [unwired: 6 in, 1 out]
          n422 = local write "Pin5"(w38) -> ()
          n423 = local read "Led 4"() -> (w37:bool)
          n424 = call-poly <vilib>:"Digital Write.vi"("Error In"=w47, "Output Value"=w37, "DO Channel"=w38, "LINX Resource"=w56) -> ("Error Out"=w46:errorcluster, "LINX Resource"=w55:T1)  [unwired: 6 in]
          n425 = call-poly <vilib>:"Digital Read.vi"("Error In"=w46, "DI Channel"=u8 6, "LINX Resource"=w55) -> ("Error Out"=w45:errorcluster, "LINX Resource"=w54:T1)  [unwired: 6 in, 1 out]
          n426 = local write "Pin6"(w35) -> ()
          n427 = local read "Led 5"() -> (w36:bool)
          n428 = call-poly <vilib>:"Digital Write.vi"("Error In"=w45, "Output Value"=w36, "DO Channel"=w35, "LINX Resource"=w54) -> ("Error Out"=w33:errorcluster, "LINX Resource"=w34:T1)  [unwired: 6 in]
        }
        n429 = local write "Tab Control"(enum32{"Inicio", "Sistema"}."Sistema" ("Tab Control")) -> ()
        n430 = call <vilib>:"Close.vi"("Error In"=w19, "LINX Resource"=w20) -> ("Error Out"=w27:errorcluster)  [unwired: 9 in]
        n431 = call <vilib>:"Simple Error Handler.vi"("error in (no error)"=w27) -> ()  [unwired: 4 in, 5 out]
        "Contenido" <- 0.0 ("Contenido")
        "Pin2" <- 0.0 ("Pin2")
        "Pin3" <- 0.0 ("Pin3")
        "Pin4" <- 0.0 ("Pin4")
        "Pin5" <- 0.0 ("Pin5")
        "Pin6" <- 0.0 ("Pin6")
      }
      frame #2 {
        n432 = local write "Tab Control"(enum32{"Inicio", "Sistema"}."Inicio" ("Tab Control")) -> ()
      }
    }
  }
  n433 = local write "Usuario"("" ("Usuario")) -> ()
  n434 = local write "Contraseña"("" ("Contraseña")) -> ()
